vi "ScintComb2HistClustIndex.vi"(10 "Secondary":i32, 11 "Primary":i32) -> (3 "Numeric":i32)   [LabVIEW 2016]
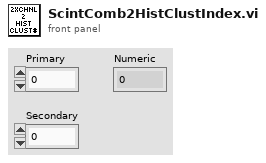
[diagram p1: front panel]
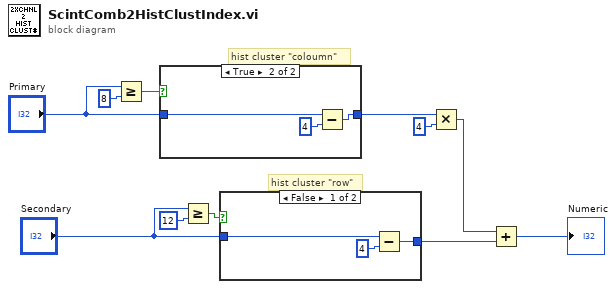
[diagram p0: block diagram]
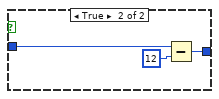
[diagram p2: hidden frame]
diagram:
  # "hist cluster \"row\""
  # "hist cluster \"coloumn\""
  n1 = Greater Or Equal?(x="Primary", y=8) -> (x >= y?=w2:bool)
  n2 = case shown="True" w2 {
    tunnel: "Primary" -> [w12 w15]
    tunnel: [w12 w13] -> w7
    frame False {
    }
    frame True {
      n3 = Subtract(x=w15, y=4) -> (x-y=w13:i32)
    }
  }
  n4 = Greater Or Equal?(x="Secondary", y=12) -> (x >= y?=w5:bool)
  n5 = case shown="False" w5 {
    tunnel: "Secondary" -> [w18 w21]
    tunnel: [w16 w19] -> w10
    frame False {
      n6 = Subtract(x=w18, y=4) -> (x-y=w16:i32)
    }
    frame True {
      n7 = Subtract(x=w21, y=12) -> (x-y=w19:i32)
    }
  }
  n8 = Multiply(x=w7, y=4) -> (x*y=w9:i32)
  n9 = Add(x=w9, y=w10) -> (x+y=→"Numeric":i32)
